vi "ProcessCalibrationData_Striptest.vi"(5 "Sensor Type":string, 10 "Fiducial 2":dbl[][](array[numeric]) format="%#_8g", 11 "Fiducial 1":dbl[][](array[numeric]) format="%#_8g") -> (2 "Avg Length":dbl format="%0.2f")   [LabVIEW 2019]
uses:
  <vilib>/Analysis/baseanly.llb/Mean (DBL).vi
  <vilib>/Analysis/NI_AALBase.lvlib
panel:
  # "Here a table of the co-ordinates for each interation of finding the fiducial can be found. Useful for debugging."
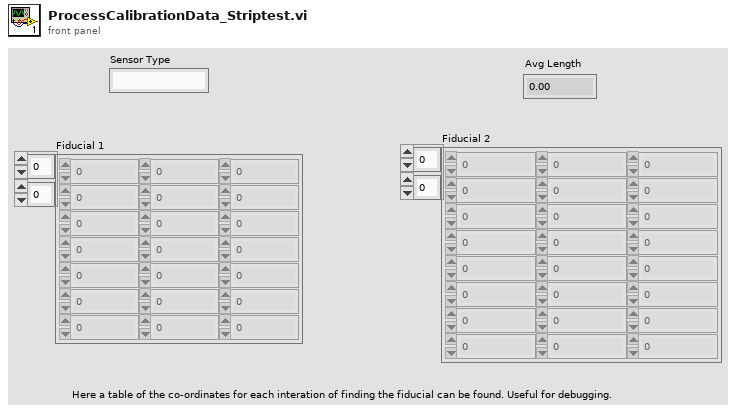
[diagram p1: front panel]
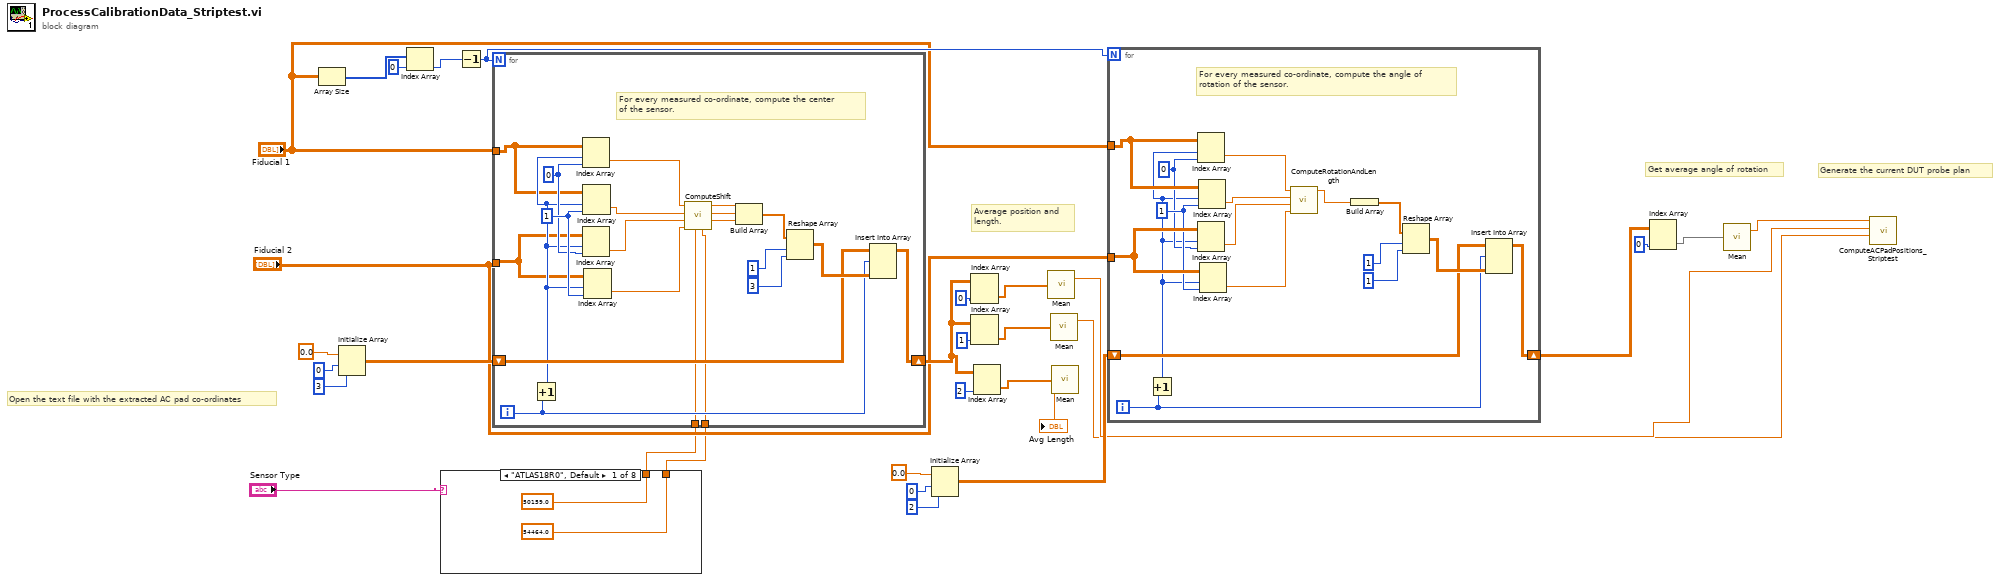
[diagram p0: block diagram]
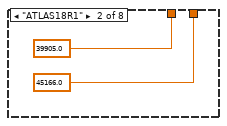
[diagram p2: hidden frame]
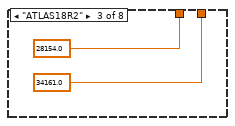
[diagram p3: hidden frame]
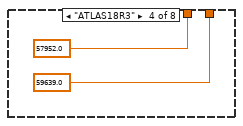
[diagram p4: hidden frame]
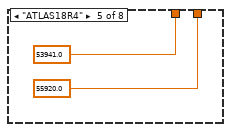
[diagram p5: hidden frame]
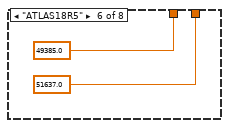
[diagram p6: hidden frame]
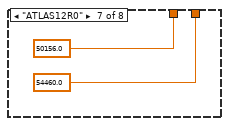
[diagram p7: hidden frame]
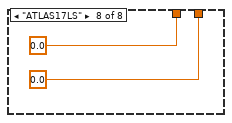
[diagram p8: hidden frame]
diagram:
  # "Generate the current DUT probe plan"
  # "Get average angle of rotation"
  # "Average position and\nlength."
  # "Open the text file with the extracted AC pad co-ordinates"
  n1 = Array Size(array="Fiducial 1") -> (size(s)=w28:i32[])
  n2 = Initialize Array(0.0 ("element"), 0 ("dimension size"), 3 ("dimension size")) -> (w26:dbl[][])
  n3 = Index Array(array=w28, index=0) -> (element=w24:i32)
  n4 = case shown="\"ATLAS18R0\", Default" "Sensor Type" {
    tunnel: [50159.0 39905.0 28154.0 57952.0 53941.0 49385.0 50156.0 0.0] -> w6
    tunnel: [54464.0 45166.0 34161.0 59639.0 55920.0 51637.0 54460.0 0.0] -> w5
    frame "ATLAS18R0", Default {
    }
    frame "ATLAS18R1" {
    }
    frame "ATLAS18R2" {
    }
    frame "ATLAS18R3" {
    }
    frame "ATLAS18R4" {
    }
    frame "ATLAS18R5" {
    }
    frame "ATLAS12R0" {
    }
    frame "ATLAS17LS" {
    }
  }
  n5 = Decrement(x=w24) -> (x-1=w14:i32)
  n6 = for {
    N: w14 -> [_]
    tunnel: "Fiducial 1" -> [w58]
    tunnel: "Fiducial 2" -> [w57]
    shift-right: [w62] -> w12
    shift-left: w26 -> [w61]
    tunnel: w6 -> [w49]
    tunnel: w5 -> [w48]
    i -> [w63]
    w68 = 1 ("disabled index (col)")
    w67 = 0 ("disabled index (col)")
    # "For every measured co-ordinate, compute the center\nof the sensor."
    n7 = Increment(x=w63) -> (x+1=w59:i32)
    n8 = Index Array(array=w58, index (row)=w59, index (col)=w67) -> (element=w53:dbl)
    n9 = Index Array(array=w57, index (row)=w59, index (col)=w67) -> (element=w55:dbl)
    n10 = Index Array(array=w58, index (row)=w59, index (col)=w68) -> (element=w54:dbl)
    n11 = Index Array(array=w57, index (row)=w59, index (col)=w68) -> (element=w56:dbl)
    n12 = call "ComputeShift.vi"("X1"=w53, "Y1"=w54, "X2"=w55, "Y2"=w56, "Dist Right"=w49, "Dist Left"=w48) -> ("XShift"=w52:dbl, "YShift"=w51:dbl, "Length"=w50:dbl)  [unwired: 2 in]
    n13 = Build Array(w52, w51, w50) -> (w65:dbl[])
    n14 = Reshape Array(w65, 1 ("dimension size"), 3 ("dimension size")) -> (w66:dbl[][])
    n15 = Insert Into Array(array=w61, index (row)=w63, new element=w66) -> (w62:dbl[][])  [unwired: 1 in]
  }
  n16 = Initialize Array(0.0 ("element"), 0 ("dimension size"), 2 ("dimension size")) -> (w15:dbl[][])
  n17 = Index Array(array=w12, index (col)=0 ("disabled index (col)")) -> (element=w23:dbl[])  [unwired: 1 in]
  n18 = Index Array(array=w12, index (col)=1 ("disabled index (col)")) -> (element=w22:dbl[])  [unwired: 1 in]
  n19 = Index Array(array=w12, index (col)=2 ("disabled index (col)")) -> (element=w10:dbl[])  [unwired: 1 in]
  n20 = call-poly <vilib>:"Mean.vi"("X"=w23) -> ("mean"=w2:dbl)  [unwired: 1 out]
  n21 = call-poly <vilib>:"Mean.vi"("X"=w22) -> ("mean"=w1:dbl)  [unwired: 1 out]
  n22 = call-poly <vilib>:"Mean.vi"("X"=w10) -> ("mean"=→"Avg Length":dbl)  [unwired: 1 out]
  n23 = for {
    N: w14 -> [_]
    tunnel: "Fiducial 1" -> [w85]
    tunnel: "Fiducial 2" -> [w84]
    shift-right: [w77] -> w13
    shift-left: w15 -> [w76]
    i -> [w78]
    w83 = 1 ("disabled index (col)")
    w82 = 0 ("disabled index (col)")
    # "For every measured co-ordinate, compute the angle of \nrotation of the sensor."
    n24 = Increment(x=w78) -> (x+1=w74:i32)
    n25 = Index Array(array=w85, index (row)=w74, index (col)=w82) -> (element=w73:dbl)
    n26 = Index Array(array=w84, index (row)=w74, index (col)=w82) -> (element=w71:dbl)
    n27 = Index Array(array=w85, index (row)=w74, index (col)=w83) -> (element=w72:dbl)
    n28 = Index Array(array=w84, index (row)=w74, index (col)=w83) -> (element=w70:dbl)
    n29 = call "ComputeRotationAndLength.vi"("Y2"=w70, "X2"=w71, "Y1"=w72, "X1"=w73) -> ("Theta (Rad)"=w69:dbl)  [unwired: 7 in]
    n30 = Build Array(w69) -> (w80:dbl[])
    n31 = Reshape Array(w80, 1 ("dimension size"), 1 ("dimension size")) -> (w81:dbl[][])
    n32 = Insert Into Array(array=w76, index (row)=w78, new element=w81) -> (w77:dbl[][])  [unwired: 1 in]
  }
  n33 = Index Array(array=w13, index (col)=0 ("disabled index (col)")) -> (element=w19:dbl[])  [unwired: 1 in]
  n34 = call-poly <vilib>:"Mean.vi"("X"=w19) -> ("mean"=w3:dbl)  [unwired: 1 out]
  n35 = call "ComputeACPadPositions_Striptest.vi"("Theta Calibration"=w3, "X cp"=w2, "Y cp"=w1) -> ()  [unwired: 8 in]
